vi "Recursive Merge.vi"(7 "$Path or Item Name":string, 8 "error in (no error)":errorcluster, 9 "JSON Object to Merge":string, 11 "JSON Schema in":string) -> (0 "error out":errorcluster, 3 "JSON Schema out":string)   [LabVIEW 2019, in "JSON-Schema.lvlib"]
uses:
  JSON-Schema.lvlib
  <vilib>/JDP Science/JSONtext/Next JSON Value.vi
  <vilib>/JDP Science/JSONtext/String Subset.vi
  <vilib>/JDP Science/JSONtext/Parsing/Advance past next JSON Value (inlined COPY).vi
  <vilib>/JDP Science/JSONtext/Parsing/Advance past whitespace.vi
  <vilib>/JDP Science/JSONtext/Parsing/Advance past String.vi
  <vilib>/JDP Science/JSONtext/Parsing/Advance past Number.vi
  <vilib>/JDP Science/JSONtext/Parsing/Advance past Line Ending.vi
  <vilib>/JDP Science/JSONtext/Parsing/Parse Full Path or Item Name.vi
  <vilib>/JDP Science/JSONtext/Parsing/Advance past Array.vi
  <vilib>/JDP Science/JSONtext/Parsing/Advance past Object.vi
  <vilib>/JDP Science/JSONtext/support/Error Cluster From Code.vi
  <vilib>/JDP Science/JSONtext/Offset/Find Item Locations by Path.vi
  <vilib>/JDP Science/JSONtext/JSONtext.lvlib
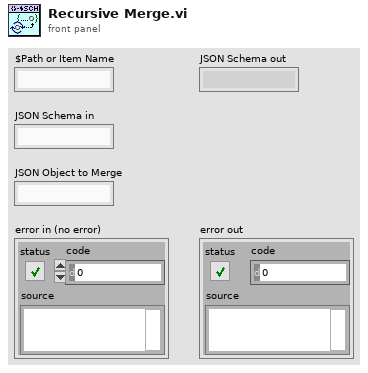
[diagram p1: front panel]
types:
  T1 = typedef "JSONtext.lvlib/JSON Value Type.ctl" = enum16{"Not a JSON Value", "JSON Object", "JSON Array", "String", "Number", "true", "false", "null"}
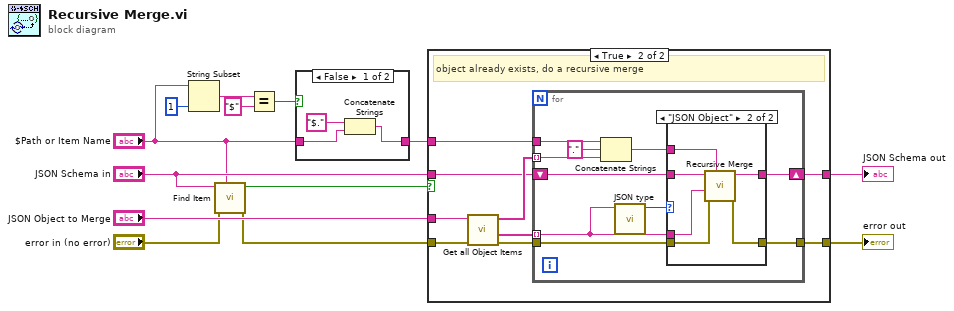
[diagram p0: block diagram]
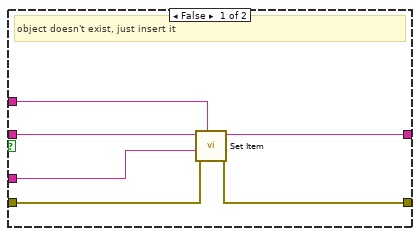
[diagram p3: hidden frame]
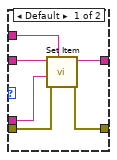
[diagram p4: hidden frame]
diagram:
  n1 = String Subset(string="$Path or Item Name", length (rest)=1 ("length (rest)")) -> (substring=w10:string)  [unwired: 1 in]
  n2 = call <vilib>:"Find Item.vi"("$Path or Item Name"="$Path or Item Name", "error in (no error)"="error in (no error)", "JSON"="JSON Schema in") -> ("error out"=w6:errorcluster, "Found"=w4:bool)  [unwired: 5 in, 2 out]
  n3 = Equal?(x=w10, y="$") -> (x = y?=w3:bool)
  n4 = case shown="False" w3 {
    tunnel: "$Path or Item Name" -> [w14 w17]
    tunnel: [w15 w17] -> w1
    frame False {
      n5 = Concatenate Strings("$." ("string"), w14) -> (w15:string)
    }
    frame True {
    }
  }
  n6 = case shown="True" w4 {
    tunnel: [w21 w31] -> w13
    tunnel: "JSON Object to Merge" -> [w23 w29]
    tunnel: [w20 w28] -> w11
    tunnel: w1 -> [w19 w26]
    tunnel: w6 -> [w22 w25]
    tunnel: "JSON Schema in" -> [w18 w24]
    frame False {
      # "object doesn't exist, just insert it"
      n7 = call <vilib>:"Set Item.vi"("$Path or Item Name"=w19, "error in (no error)"=w22, "JSON to Insert"=w23, "JSON"=w18) -> ("error out"=w21:errorcluster, "<JSON>"=w20:string)  [unwired: 4 in, 1 out]
    }
    frame True {
      # "object already exists, do a recursive merge"
      n8 = call <vilib>:"Get all Object Items.vi"("error in (no error)"=w25, "JSON"=w29) -> ("error out"=w30:errorcluster, "<JSON>"=w32:string[], "Item Names"=w27:string[])  [unwired: 6 in, 1 out]
      n9 = for {
        shift-right: [w42] -> w28
        shift-left: w24 -> [w41]
        tunnel: w30 -> [w40]
        tunnel: [w39] -> w31
        tunnel: w26 -> [w38]
        tunnel: w27 -> [w37] mode=indexing
        tunnel: w32 -> [w34] mode=indexing
        n10 = Concatenate Strings(w38, "." ("string"), w37) -> (w33:string)
        n11 = call <vilib>:"JSON type.vi"("JSON"=w34) -> ("JSON Value Type"=w35:T1)  [unwired: 9 in, 1 out]
        n12 = case shown="\"JSON Object\"" w35 {
          tunnel: [w44 w50] -> w42
          tunnel: w41 -> [w47 w51]
          tunnel: w40 -> [w46 w54]
          tunnel: [w45 w53] -> w39
          tunnel: w33 -> [w48 w52]
          tunnel: w34 -> [w43 w49]
          frame Default {
            n13 = call <vilib>:"Set Item.vi"("$Path or Item Name"=w48, "error in (no error)"=w46, "JSON to Insert"=w43, "JSON"=w47) -> ("error out"=w45:errorcluster, "<JSON>"=w44:string)  [unwired: 4 in, 1 out]
          }
          frame "JSON Object" {
            n14 = call "Recursive Merge.vi"("$Path or Item Name"=w52, "error in (no error)"=w54, "JSON Object to Merge"=w49, "JSON Schema in"=w51) -> ("error out"=w53:errorcluster, "JSON Schema out"=w50:string)  [unwired: 6 in]
          }
        }
      }
    }
  }
  "error out" <- w13
  "JSON Schema out" <- w11
